vi "Normalization Controller.vi"(0 "TYPE LIST HERE -  RN;RN;RN;...   (max of 10)":string, 1 "START":bool, 2 "RETURN":bool) -> (3 "Right Ave":cluster{ext, ext}[](graph), 4 "Left Ave":cluster{ext, ext}[](graph), 5 "File Write Error":bool, 6 "Save?":bool)   [LabVIEW 2020]
panel:
  out "CAT":i32=365
  out "Runs Plotted":string
  out "Right Ear":cluster{cluster{ext, ext}[]}[](graph)
  out "Left Ear":cluster{cluster{ext, ext}[]}[](graph)
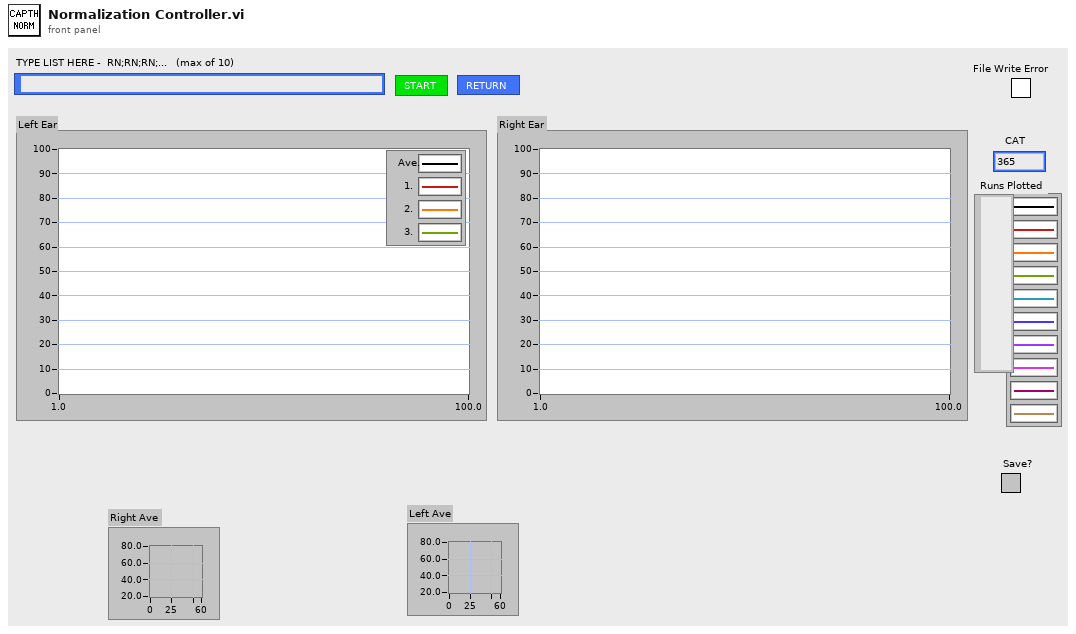
[diagram p1: front panel]
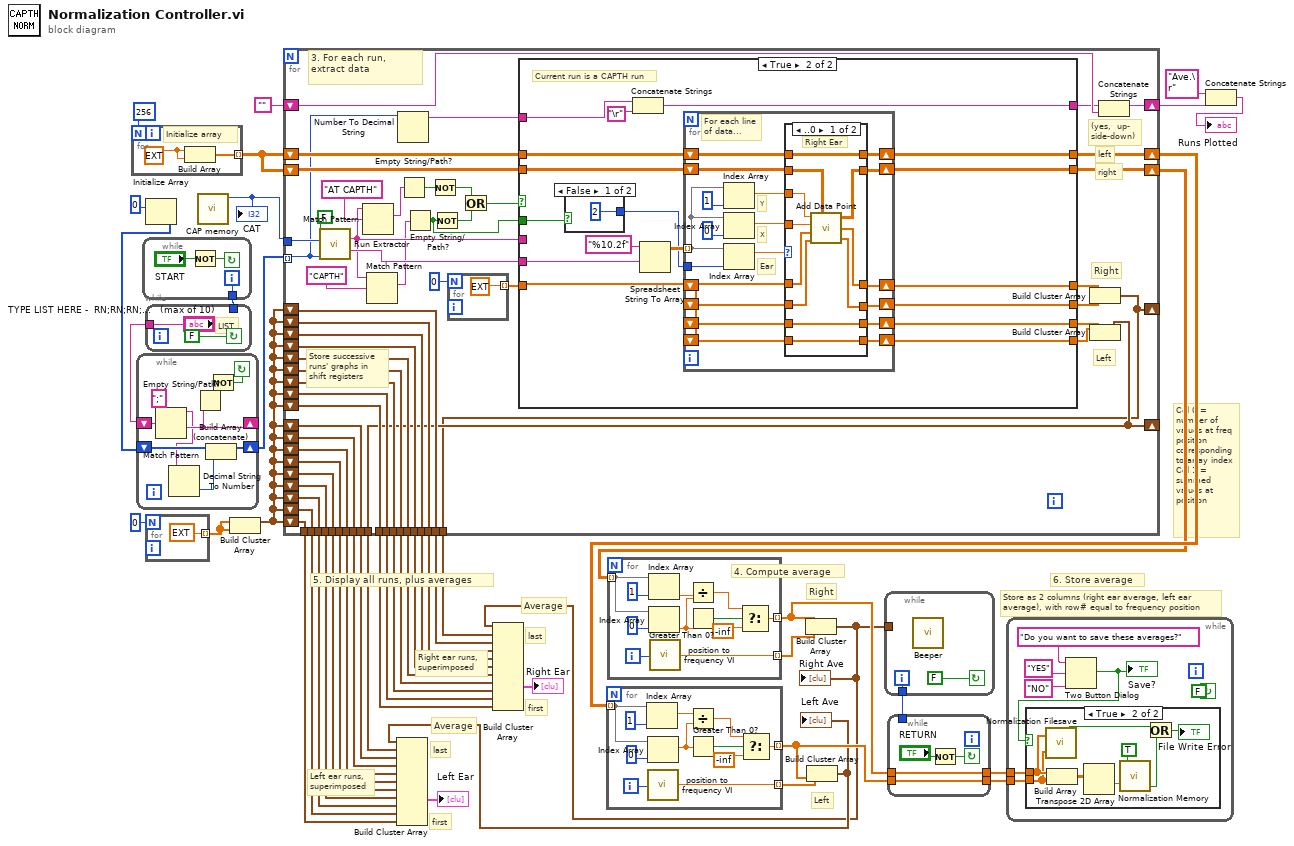
[diagram p0: block diagram]
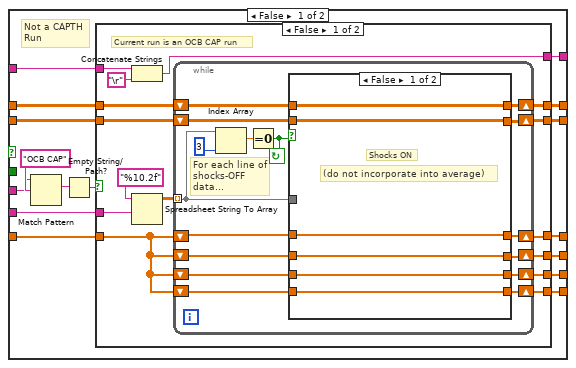
[diagram p3: hidden frame]
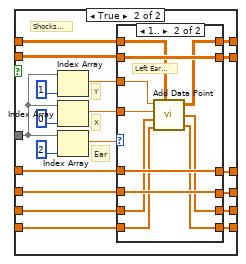
[diagram p4: hidden frame]
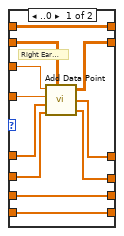
[diagram p5: hidden frame]
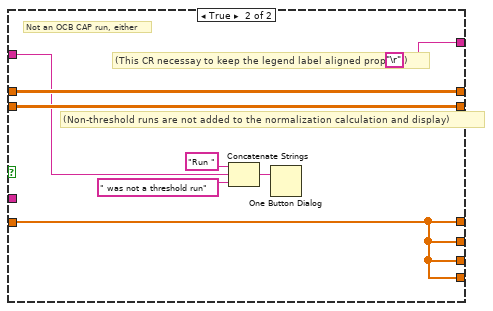
[diagram p6: hidden frame]
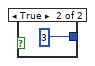
[diagram p7: hidden frame]
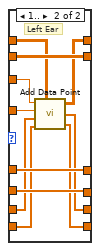
[diagram p8: hidden frame]
diagram:
  # "Average"
  # "Average"
  # "Left ear runs, superimposed"
  # "6. Store average"
  # "Store as 2 columns (right ear average, left ear average), with row# equal to frequency position"
  # "first"
  # "last"
  # "first"
  # "last"
  # "5. Display all runs, plus averages"
  # "Right ear runs, superimposed"
  # "4. Compute average"
  # "Col 0 = number of values at freq position corresponding to array index\nCol 1 = summed values at position"
  # "Right"
  # "Left"
  n1 = for {
    N: 256 -> [_]
    tunnel: [w50] -> w19 mode=indexing
    w49 = ext 0.0
    # "Initialize array"
    n2 = Build Array(w49, w49) -> (w50:ext[])
  }
  n3 = while {
    tunnel: [w51] -> w35
    i -> [w51]
    stop <- w52 continue-if-true
    n4 = Not(x="START") -> (.not. x?=w52:bool)
  }
  n5 = Initialize Array(0) -> (w3:i32[])  [unwired: 1 in]
  n6 = while {
    tunnel: ["TYPE LIST HERE -  RN;RN;RN;...   (max of 10)"] -> w4
    tunnel: w35 -> [_]
    stop <- FALSE continue-if-true
    # "LIST"
  }
  n7 = while {
    shift-left: w3 -> [w58]
    shift-right: [w64] -> w1
    shift-left: w4 -> [w63]
    shift-right: [w61] -> _
    stop <- w59 continue-if-true
    n8 = Match Pattern(string=w63, regular expression=";") -> (before substring=w57:string, after substring=w61:string)  [unwired: 1 in, 2 out]
    n9 = Decimal String To Number(string=w57) -> (number=w56:i32)  [unwired: 2 in, 1 out]
    n10 = Empty String/Path?(string/path=w61) -> (empty?=w60:bool)
    n11 = Build Array (concatenate)(w58, w56) -> (w64:i32[])
    n12 = Not(x=w60) -> (.not. x?=w59:bool)
  }
  n13 = for {
    N: 0 -> [_]
    tunnel: [ext 0.0] -> w47 mode=indexing
  }
  n14 = call "CAP memory.vi"() -> ("CN"=w36:u32)  [unwired: 6 in, 3 out]
  "CAT" <- w36
  n15 = Build Cluster Array(w47, w47) -> (w17:cluster{ext, ext}[])
  n16 = for {
    shift-right: [w87] -> w21
    shift-left: w19 -> [w90]
    shift-right: [w86] -> w18
    shift-left: w19 -> [w88]
    shift-right: [w93] -> _
    shift-left: w17 -> [w102]
    shift-left: w17 -> [w94]
    shift-left: w17 -> [w95]
    shift-left: w17 -> [w96]
    shift-left: w17 -> [w97]
    shift-left: w17 -> [w98]
    shift-left: w17 -> [w99]
    shift-left: w17 -> [w100]
    shift-left: w17 -> [w101]
    shift-right: [w81] -> w14
    shift-left: "" -> [w79]
    shift-right: [w92] -> _
    shift-left: w17 -> [w113]
    shift-left: w17 -> [w105]
    shift-left: w17 -> [w106]
    shift-left: w17 -> [w107]
    shift-left: w17 -> [w108]
    shift-left: w17 -> [w109]
    shift-left: w17 -> [w110]
    shift-left: w17 -> [w111]
    shift-left: w17 -> [w112]
    tunnel: w1 -> [w80] mode=indexing
    tunnel: [w93] -> w33
    tunnel: [w94] -> w24
    tunnel: [w95] -> w25
    tunnel: [w96] -> w26
    tunnel: [w97] -> w27
    tunnel: [w98] -> w28
    tunnel: [w99] -> w29
    tunnel: [w100] -> w30
    tunnel: [w101] -> w31
    tunnel: [w102] -> w32
    tunnel: w36 -> [w103]
    tunnel: [w92] -> w46
    tunnel: [w105] -> w37
    tunnel: [w106] -> w38
    tunnel: [w107] -> w39
    tunnel: [w108] -> w40
    tunnel: [w109] -> w41
    tunnel: [w110] -> w42
    tunnel: [w111] -> w43
    tunnel: [w112] -> w44
    tunnel: [w113] -> w45
    # "right"
    # "left"
    # "Store successive runs' graphs in shift registers"
    # "3. For each run, extract data"
    # "(yes,  up- side-down)"
    # "Left"
    # "Right"
    n17 = call "Run Extractor"("Run #"=w80, "Cat #"=w103, "CAP (F) - SINGLE UNIT (T)"=FALSE) -> ("DATA STRING"=w73:string, "HEADER STRING"=w72:string)  [unwired: 1 in, 1 out]
    n18 = Match Pattern(string=w72, regular expression="AT CAPTH") -> (match substring=w75:string)  [unwired: 1 in, 3 out]
    n19 = Match Pattern(string=w72, regular expression="CAPTH") -> (match substring=w70:string)  [unwired: 1 in, 3 out]
    n20 = Number To Decimal String(number=w80) -> (decimal integer string=w77:string)  [unwired: 1 in]
    n21 = Empty String/Path?(string/path=w75) -> (empty?=w74:bool)
    n22 = Empty String/Path?(string/path=w70) -> (empty?=w66:bool)
    n23 = Not(x=w74) -> (.not. x?=w67:bool)
    n24 = Not(x=w66) -> (.not. x?=w68:bool)
    n25 = for {
      N: 0 -> [_]
      tunnel: [ext 0.0] -> w89 mode=indexing
    }
    n26 = Or(x=w67, y=w68) -> (x .or. y?=w69:bool)
    n27 = case shown="True" w69 {
      tunnel: w72 -> [w127 _]
      tunnel: [w122 w221] -> w78
      tunnel: [w116 w222] -> w82
      tunnel: [w117 w223] -> w83
      tunnel: [w118 w224] -> w84
      tunnel: [w119 w225] -> w85
      tunnel: [w120 w226] -> w86
      tunnel: [w121 w227] -> w87
      tunnel: w77 -> [w115 w220]
      tunnel: w88 -> [w124 w228]
      tunnel: w89 -> [w123 w229]
      tunnel: w90 -> [w125 w230]
      tunnel: w73 -> [w114 w216]
      tunnel: w66 -> [_ w217]
      frame False {
        # "Not a CAPTH Run"
        n28 = Match Pattern(string=w127, regular expression="OCB CAP") -> (match substring=w129:string)  [unwired: 1 in, 3 out]
        n29 = Empty String/Path?(string/path=w129) -> (empty?=w126:bool)
        n30 = case shown="False" w126 {
          tunnel: w114 -> [w143 _]
          tunnel: w115 -> [w141 w210]
          tunnel: [w132 w212] -> w116
          tunnel: [w133 w212] -> w117
          tunnel: [w134 w212] -> w118
          tunnel: [w135 w212] -> w119
          tunnel: [w136 w213] -> w120
          tunnel: [w137 w214] -> w121
          tunnel: [w142 "\r"] -> w122
          tunnel: w123 -> [w130 w212]
          tunnel: w124 -> [w139 w213]
          tunnel: w125 -> [w140 w214]
          frame False {
            # "Current run is an OCB CAP run"
            n31 = Concatenate Strings(w141, "\r") -> (w142:string)
            n32 = Spreadsheet String To Array(format string="%10.2f", spreadsheet string=w143) -> (array=w138:dbl[][])  [unwired: 2 in]
            n33 = while {
              tunnel: w138 -> [w158] mode=indexing
              shift-left: w140 -> [w153]
              shift-right: [w151] -> w137
              shift-left: w139 -> [w152]
              shift-right: [w150] -> w136
              shift-left: w130 -> [w157]
              shift-right: [w149] -> w135
              shift-left: w130 -> [w156]
              shift-right: [w148] -> w134
              shift-left: w130 -> [w155]
              shift-right: [w147] -> w133
              shift-left: w130 -> [w154]
              shift-right: [w146] -> w132
              stop <- w145 continue-if-true
              # "For each line of shocks-OFF data..."
              n34 = Index Array(array=w158, index=3) -> (element=w160:dbl)
              n35 = Equal To 0?(x=w160) -> (x = 0?=w145:bool)
              n36 = case shown="False" w145 {
                tunnel: [w161 w167] -> w146
                tunnel: [w162 w168] -> w147
                tunnel: [w163 w169] -> w148
                tunnel: [w164 w170] -> w149
                tunnel: [w165 w171] -> w150
                tunnel: [w166 w172] -> w151
                tunnel: w154 -> [w161 w173]
                tunnel: w155 -> [w162 w174]
                tunnel: w156 -> [w163 w175]
                tunnel: w157 -> [w164 w176]
                tunnel: w152 -> [w165 w177]
                tunnel: w153 -> [w166 w178]
                tunnel: w158 -> [_ w179]
                frame False {
                  # "Shocks ON"
                  # "(do not incorporate into average)"
                }
                frame True {
                  # "Shocks OFF"
                  # "Ear"
                  # "X"
                  # "Y"
                  n37 = Index Array(array=w179, index=1) -> (element=w184:dbl)
                  n38 = Index Array(array=w179, index=0) -> (element=w185:dbl)
                  n39 = Index Array(array=w179, index=2) -> (element=w181:dbl)
                  n40 = case shown="1.." w181 {
                    tunnel: w185 -> [w191 w202]
                    tunnel: w184 -> [w192 w203]
                    tunnel: [w194 w199] -> w172
                    tunnel: w178 -> [w194 w204]
                    tunnel: [w188 w205] -> w171
                    tunnel: w177 -> [w193 w205]
                    tunnel: w173 -> [w195 w200]
                    tunnel: [w195 w197] -> w167
                    tunnel: w174 -> [w196 w201]
                    tunnel: [w196 w198] -> w168
                    tunnel: w175 -> [w189 w207]
                    tunnel: w176 -> [w190 w206]
                    tunnel: [w186 w207] -> w169
                    tunnel: [w187 w206] -> w170
                    frame ..0 {
                      # "Right Ear Data"
                      n41 = call "Add Data Point"("Y"=w192, "X"=w191, "Y Array In"=w190, "X Array In"=w189, "2D Norm Array In"=w193) -> ("2D Norm Array Out"=w188:ext[][], "Y Array Out"=w187:ext[], "X Array Out"=w186:ext[])
                    }
                    frame 1.. {
                      # "Left Ear Data"
                      n42 = call "Add Data Point"("Y"=w203, "X"=w202, "Y Array In"=w201, "X Array In"=w200, "2D Norm Array In"=w204) -> ("2D Norm Array Out"=w199:ext[][], "Y Array Out"=w198:ext[], "X Array Out"=w197:ext[])
                    }
                  }
                }
              }
            }
          }
          frame True {
            # "Not an OCB CAP run, either"
            # "(Non-threshold runs are not added to the normalization calculation and display)"
            # "(This CR necessay to keep the legend label aligned properly)"
            n43 = Concatenate Strings("Run ", w210, " was not a threshold run") -> (w208:string)
            n44 = One Button Dialog(message=w208) -> ()  [unwired: 1 in, 1 out]
          }
        }
      }
      frame True {
        # "Current run is a CAPTH run"
        n45 = case shown="False" w217 {
          tunnel: [2 3] -> w218
          frame False {
          }
          frame True {
          }
        }
        n46 = Concatenate Strings(w220, "\r") -> (w221:string)
        n47 = Spreadsheet String To Array(format string="%10.2f", spreadsheet string=w216) -> (array=w232:dbl[][])  [unwired: 2 in]
        n48 = for {
          shift-right: [w243] -> w227
          shift-left: w230 -> [w244]
          shift-right: [w241] -> w226
          shift-left: w228 -> [w242]
          shift-right: [w245] -> w222
          shift-left: w229 -> [w246]
          shift-right: [w247] -> w223
          shift-left: w229 -> [w248]
          shift-right: [w252] -> w224
          shift-left: w229 -> [w249]
          shift-right: [w251] -> w225
          shift-left: w229 -> [w250]
          tunnel: w232 -> [w238] mode=indexing
          tunnel: w218 -> [w235]
          # "X"
          # "Y"
          # "Ear"
          # "For each line of data..."
          n49 = Index Array(array=w238, index=1) -> (element=w236:dbl)
          n50 = Index Array(array=w238, index=0) -> (element=w237:dbl)
          n51 = Index Array(array=w238, index=w235) -> (element=w253:dbl)
          n52 = case shown="..0" w253 {
            tunnel: w237 -> [w259 w270]
            tunnel: w236 -> [w260 w271]
            tunnel: [w262 w267] -> w243
            tunnel: w244 -> [w262 w272]
            tunnel: [w256 w273] -> w241
            tunnel: w242 -> [w261 w273]
            tunnel: w246 -> [w263 w268]
            tunnel: [w263 w265] -> w245
            tunnel: w248 -> [w264 w269]
            tunnel: [w264 w266] -> w247
            tunnel: w249 -> [w257 w275]
            tunnel: w250 -> [w258 w274]
            tunnel: [w254 w275] -> w252
            tunnel: [w255 w274] -> w251
            frame ..0 {
              # "Right Ear"
              n53 = call "Add Data Point"("Y"=w260, "X"=w259, "Y Array In"=w258, "X Array In"=w257, "2D Norm Array In"=w261) -> ("2D Norm Array Out"=w256:ext[][], "Y Array Out"=w255:ext[], "X Array Out"=w254:ext[])
            }
            frame 1.. {
              # "Left Ear"
              n54 = call "Add Data Point"("Y"=w271, "X"=w270, "Y Array In"=w269, "X Array In"=w268, "2D Norm Array In"=w272) -> ("2D Norm Array Out"=w267:ext[][], "Y Array Out"=w266:ext[], "X Array Out"=w265:ext[])
            }
          }
        }
      }
    }
    n55 = Build Cluster Array(w84, w85) -> (w92:cluster{ext, ext}[])
    n56 = Build Cluster Array(w82, w83) -> (w93:cluster{ext, ext}[])
    n57 = Concatenate Strings(w78, w79) -> (w81:string)
  }
  n58 = for {
    tunnel: [w278] -> w11 mode=indexing
    tunnel: [w282] -> w22 mode=indexing
    tunnel: w21 -> [w285] mode=indexing
    i -> [w283]
    n59 = Index Array(array=w285, index=1) -> (element=w284:ext)
    n60 = Index Array(array=w285, index=0) -> (element=w280:ext)
    n61 = call "position to frequency VI"("position"=w283) -> ("frequency"=w282:ext)
    n62 = Divide(x=w284, y=w280) -> (x/y=w279:ext)
    n63 = Greater Than 0?(x=w280) -> (x > 0?=w281:bool)
    n64 = Select(t=w279, s=w281, f=-inf) -> (s? t:f=w278:ext)
  }
  n65 = for {
    tunnel: w18 -> [w293] mode=indexing
    tunnel: [w294] -> w9 mode=indexing
    tunnel: [w288] -> w6 mode=indexing
    i -> [w295]
    n66 = Index Array(array=w293, index=1) -> (element=w296:ext)
    n67 = Index Array(array=w293, index=0) -> (element=w290:ext)
    n68 = call "position to frequency VI"("position"=w295) -> ("frequency"=w294:ext)
    n69 = Divide(x=w296, y=w290) -> (x/y=w289:ext)
    n70 = Greater Than 0?(x=w290) -> (x > 0?=w291:bool)
    n71 = Select(t=w289, s=w291, f=-inf) -> (s? t:f=w288:ext)
  }
  n72 = Build Cluster Array(w9, w6) -> (w5:cluster{"frequency":ext, ext}[])
  "Right Ave" <- w5
  n73 = Build Cluster Array(w5, w46, w45, w44, w43, w42, w41, w40, w39, w38, w37) -> (→"Right Ear":cluster{cluster{"frequency":ext, ext}[]}[])
  n74 = Build Cluster Array(w22, w11) -> (w8:cluster{"frequency":ext, ext}[])
  "Left Ave" <- w8
  n75 = Build Cluster Array(w8, w33, w32, w31, w30, w29, w28, w27, w26, w25, w24) -> (→"Left Ear":cluster{cluster{"frequency":ext, ext}[]}[])
  n76 = while {
    tunnel: [w300] -> w7
    tunnel: w5 -> [_]
    i -> [w300]
    stop <- FALSE continue-if-true
    n77 = call "Beeper"() -> ()  [unwired: 1 in]
  }
  n78 = while {
    tunnel: w11 -> [w302]
    tunnel: [w302] -> w12
    tunnel: [w301] -> w10
    tunnel: w6 -> [w301]
    tunnel: w7 -> [_]
    stop <- w303 continue-if-true
    n79 = Not(x="RETURN") -> (.not. x?=w303:bool)
  }
  n80 = while {
    tunnel: w12 -> [w308]
    tunnel: w10 -> [w307]
    stop <- FALSE continue-if-true
    n81 = Two Button Dialog(message="Do you want to save these averages?", 1:"NO", 2:"YES") -> (T button?=w306:bool)
    "Save?" <- w306
    n82 = case shown="True" w306 {
      tunnel: w307 -> [_ w316]
      tunnel: w308 -> [_ w315]
      frame False {
      }
      frame True {
        n83 = call "Normalization Filesave"("Array In Left"=w315, "Array In Right"=w316) -> ("File Error"=w313:bool)
        n84 = Build Array(w316, w315) -> (w318:ext[][])
        n85 = Transpose 2D Array(2D array=w318) -> (transposed array=w317:ext[][])
        n86 = call "Normalization Memory.vi"("Read(F) or Write(T)"=TRUE, "Array In"=w317) -> ("File Error"=w319:bool)  [unwired: 2 out]
        n87 = Or(x=w313, y=w319) -> (x .or. y?=→"File Write Error":bool)
      }
    }
  }
  n88 = Concatenate Strings("Ave.\r", w14) -> (→"Runs Plotted":string)
